vi "ATSpectrograph_monitorCommand_stopAllAxes.vi"(8 "error in (no error)":errorcluster, 11 "command_stopAllAxes_Ctl":T1) -> (0 "error out":errorcluster, 2 "function return":i32, 3 "command_stopAllAxes_Ctl out":T1)   [LabVIEW 2016, in "SALLV_ATSpectrograph.lvlib"]
doc: "int ATSpectrograph_shm_monitorCommand_stopAllAxesLV(ATSpectrograph_command_stopAllAxesLV *command_stopAllAxes_Ctl );"
uses:
  SALLV_ATSpectrograph.lvlib
  DataTypes/command_stopAllAxes.ctl
  SALLV_ATSpectrograph.so
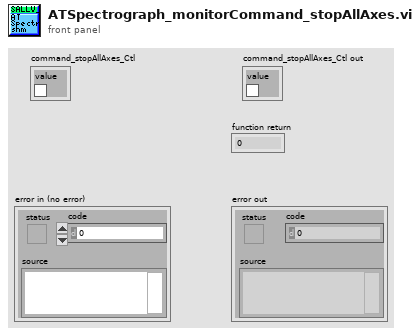
[diagram p1: front panel]
types:
  T1 = typedef "SALLV_ATSpectrograph.lvlib/command_stopAllAxes.ctl" = cluster{"value":bool}
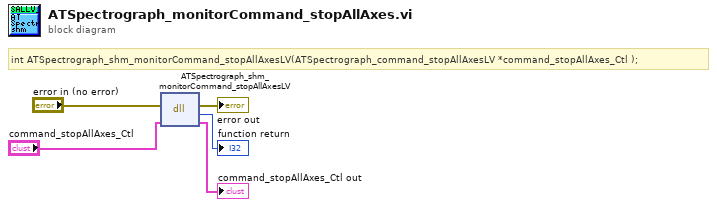
[diagram p0: block diagram]
diagram:
  # "int ATSpectrograph_shm_monitorCommand_stopAllAxesLV(ATSpectrograph_command_stopAllAxesLV *command_stopAllAxes_Ctl );"
  n1 = dll-call lib="home/harini/TCS/develop/SALLV_ATSpectrograph/SALLV_ATSpectrograph.*" fn="ATSpectrograph_shm_monitorCommand_stopAllAxesLV"(error in="error in (no error)", "command_stopAllAxes_Ctl"="command_stopAllAxes_Ctl") -> (error out=→"error out":errorcluster, →"function return":i32, "command_stopAllAxes_Ctl"=→"command_stopAllAxes_Ctl out":T1)  [unwired: 2 in, 1 out]
